vi "Yokogawa WT300 Series Measure Normal.vi"() -> ()   [LabVIEW 2016]
doc: "This example shows how to use ranging configuration and measure the normal numeric data."
uses:
  Public/Utility/Function/Create Function String (Voltage).vi
  Public/Data/Read Measurement (Normal).vi
  Yokogawa WT300 Series.lvlib
panel:
  in  "Element (1: 1)":i32(ring)=1 items=["1"=1, "2"=2, "3"=3, "Sigma A"=4]
  in  "Function (0: U)":i32(ring) items=["U", "UPPeak", "UMPeak"]
  out "Function":string
  out "Measurement":dbl
  in  "Item (1)":i32=1 min=1 max=255 step=1
  in  "Timeout (10000 ms)":i32=10000 min=1
  in  "VISA resource name":refnum<visa-resource-name>
  # "(c) 2013 Yokogawa Meters & Instruments Corporation.  All rights reserved."
  # "WT300 SERIES POWER ANALYZER"
  # "ms"
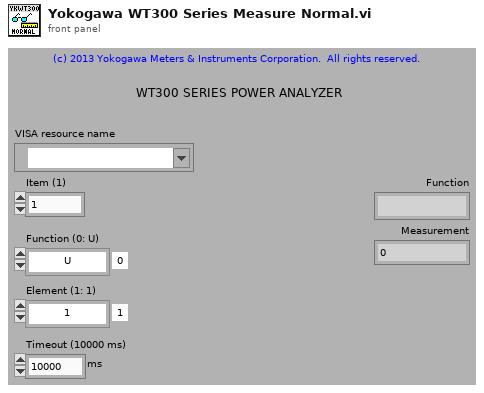
[diagram p1: front panel]
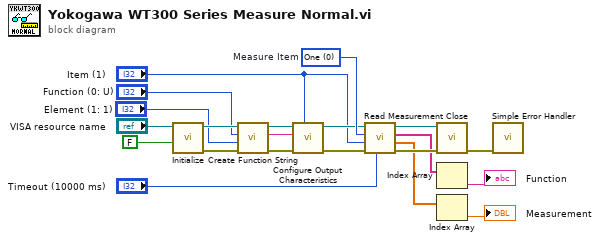
[diagram p0: block diagram]
diagram:
  w16 = 0 items=["One", "Plural"]  # Measure Item
  n1 = call "Initialize.vi"("Reset (True)"=FALSE ("Reset? (True)"), "VISA resource name"="VISA resource name") -> ("error out"=w12:errorcluster, "VISA resource name out"=w13:refnum<visa-resource-name>)  [unwired: 7 in, 1 out]
  n2 = call-poly "Create Function String.vi"("error in (no error)"=w12, "Element (1: 1)"="Element (1: 1)", "Function (0: U)"="Function (0: U)", "VISA resource name"=w13) -> ("error out"=w10:errorcluster, "Function String"=w3:string, "VISA resource name out"=w11:refnum<visa-resource-name>)  [unwired: 5 in]
  n3 = call "Configure Output Characteristics.vi"("Item (1)"="Item (1)", "error in (no error)"=w10, "Function (Empty)"=w3, "VISA resource name"=w11) -> ("error out"=w14:errorcluster, "VISA resource name out"=w15:refnum<visa-resource-name>)  [unwired: 6 in]
  n4 = call-poly "Read Measurement.vi"("Timeout (10000 ms)"="Timeout (10000 ms)", "error in (no error)"=w14, "Number of Item (15)"="Item (1)", "Measure Item (1: Plural)"=w16, "VISA resource name"=w15) -> ("error out"=w18:errorcluster, "Measurement"=w9:dbl[], "Function"=w5:string[], "VISA resource name out"=w19:refnum<visa-resource-name>)  [unwired: 3 in]
  n5 = call "Close.vi"("error in (no error)"=w18, "VISA resource name"=w19) -> ("error out"=w21:errorcluster)  [unwired: 9 in]
  n6 = Index Array(array=w5) -> (element=→"Function":string)  [unwired: 1 in]
  n7 = Index Array(array=w9) -> (element=→"Measurement":dbl)  [unwired: 1 in]
  n8 = call <vilib>:"Simple Error Handler.vi"("error in (no error)"=w21) -> ()  [unwired: 4 in, 5 out]
